vi "Get Device Name.vi"(0 "Session Handle in":T1, 11 "error in (no error)":errorcluster) -> (4 "Session Handle out":T1, 6 "device":refnum<k21>, 15 "error out":errorcluster)   [LabVIEW 2015, in "SLSC Switch.lvlib" / "SLSC Session.lvclass"]
uses:
  SLSC Session.lvclass
  Typedefs/Session Handle.ctl
  SLSC Session.lvclass/SLSC Session.ctl
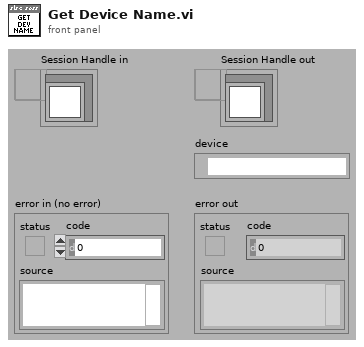
[diagram p1: front panel]
types:
  T1 = typedef "SLSC Switch.lvlib/SLSC Session.lvclass/Session Handle.ctl" = refnum<data-value>
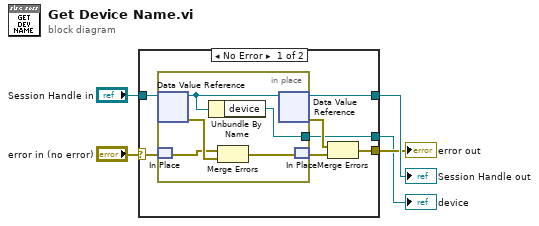
[diagram p0: block diagram]
diagram:
  n1 = case shown="No Error" "error in (no error)" {
    selector: "error in (no error)" -> [w7 w18]
    tunnel: "Session Handle in" -> [w12 w19]
    tunnel: [w11 w19] -> w4
    tunnel: [w8 w18] -> w3
    tunnel: [w6 _] -> w1
    frame No Error {
      n2 = in-place {
        in-place-border: [w13] -> w6
        n3 = in-place-dvr #1(w12) -> (w14:refnum<class "SLSC Session.lvclass">, w16:errorcluster)
        n4 = in-place-match #2(w7) -> (w15:errorcluster)
        n5 = Unbundle By Name(w14) -> ("device"=w13:refnum<k21>)
        n6 = Merge Errors(w15, w16) -> (w17:errorcluster)
        n7 = in-place-dvr #1(w14) -> (w11:T1, w9:errorcluster)
        n8 = in-place-match #2(w17) -> (w10:errorcluster)
      }
      n9 = Merge Errors(w9, w10) -> (w8:errorcluster)
    }
    frame Error {
    }
  }
  "Session Handle out" <- w4
  "error out" <- w3
  "device" <- w1
